vi "RC_Test.vi"() -> ()   [LabVIEW 2013]
uses:
  Data/TypeDefs/DynamixelCycleTracker.ctl
  Data/TypeDefs/Rudder Set Suggestions.ctl
  Data/TypeDefs/HindbrainControlOptions.ctl
  Data/TypeDefs/MotorSetup.ctl
  Data/TypeDefs/DynamixelSetupInfo.ctl
  <vilib>/FPGAPlugInAG/myRIO-1900/niLvFpga_Open_myRIO-1900.vi
  <vilib>/rvi/interface/common/dynamic/niFpgaDynamicAddResources.vi
  <vilib>/rvi/interface/nirviOpenFPGA/nirviOpenFPGA.xnode
  FPGA Bitfiles/AutonomousSailbo_FPGATarget_myRIOPWMDecoder_0snwDOwOU4s.lvbitx
  FPGA_Code/myRIO_PWM_Decoder.vi
  <instrlib>/Dynamixel Motor/Dynamixel Motor.lvlib
panel:
  out "Waveform Chart, Sail 1":dbl(graph)
  out "Waveform Chart, Sail 2":dbl(graph)
  out "error out":errorcluster[](array[cluster])
  in  "Sail 1 Calibration Speed":dbl
  in  "Sail 2 Bound Offset":dbl=800.0
  in  "Sail 1 Bound Offset":dbl=800.0
  in  "Sail 2 Calibration Speed":dbl
  in  "Use Speed\nControl":bool
  out "Position Sail 2":dbl
  out "Position Sail 1":dbl
  out "Calibration loop counter":i32
  in  "Dynamixel Bounds":T1={"Main Dynamixel Set Data"={"Lower Winch Bound (deg)"=0.0, "Upper Winch Bound (deg)"=0.0}, "Rudder Dynamixel Set Data"={"Lower Winch Bound (deg)"=15.0, "Upper Winch Bound (deg)"=60.0}, "Jib Dynamixel Set Data"={"Lower Winch Bound (deg)"=0.0, "Upper Winch Bound (deg)"=0.0}}
  in  "Sail 1 Lower Bound":dbl
  in  "Sail 2 Lower Bound":dbl
  in  "Stop Calibration":bool
  in  "Mode control":T3=enum."RC_control"
  out "Motors IDs Found":u8[](array[numeric])
  out "Commanded rudder value":T4 min=-0.95 max=0.95 scale=1.0..-1.0
  out "Commanded sail value":dbl
  out "Write loop counter":i32
  out "Updated Dynamixel Cycles":T5
  out "Dynamixel Positions (deg)":dbl[](array[numeric])
  out "Read loop counter":i32
  in  "Stop reading":bool
  in  "Stop writing":bool
  in  "VISA resource name":refnum<visa-resource-name>="ASRL3::INSTR"
  # "Read from RC Controller"
  # "Read from Dynamixels"
  # "Check value rudder is being commanded to in position control"
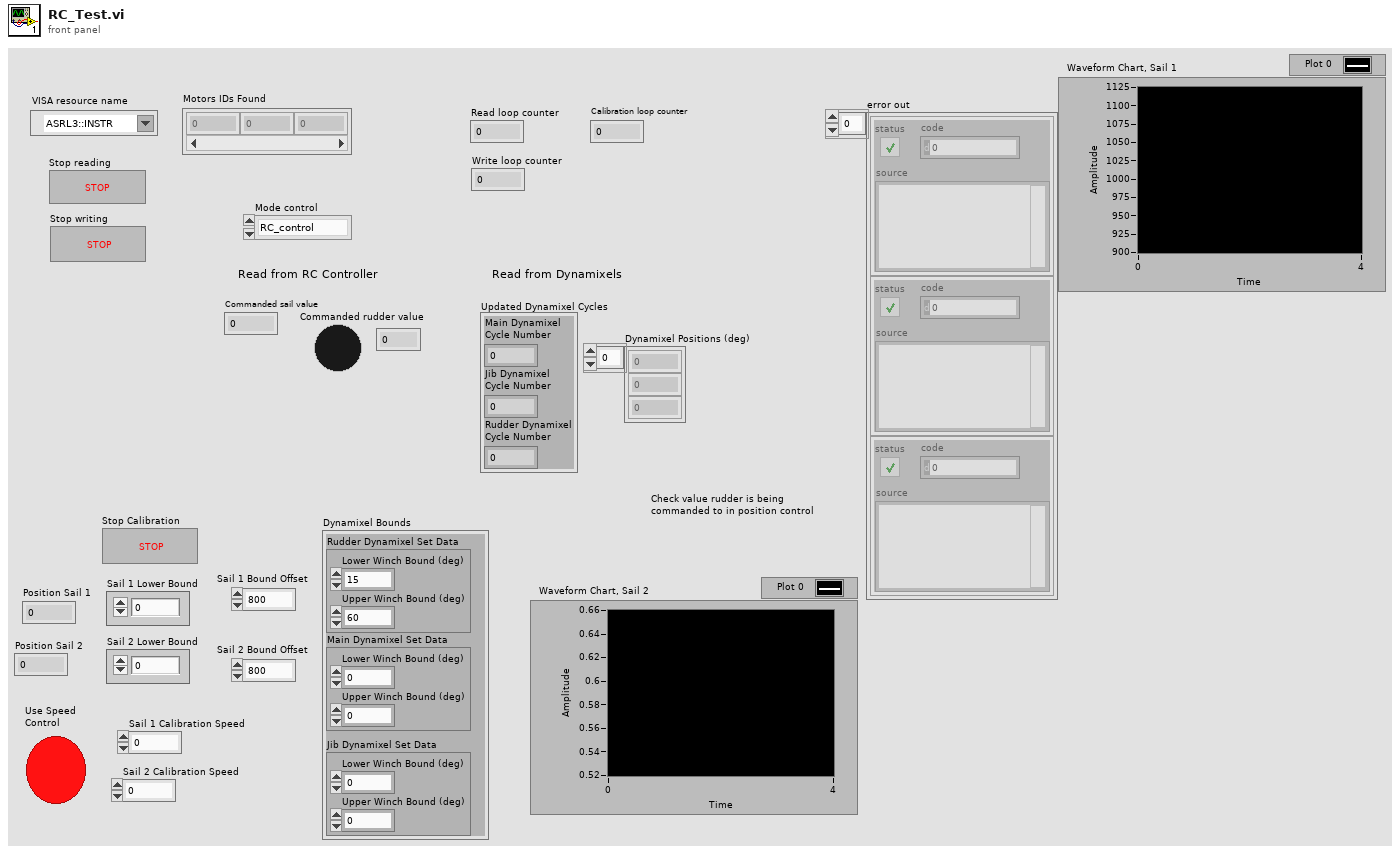
[diagram p1: front panel]
types:
  T1 = typedef "MotorSetup.ctl" = cluster{"Main Dynamixel Set Data":T2, "Rudder Dynamixel Set Data":T2, "Jib Dynamixel Set Data":T2}
  T2 = typedef "DynamixelSetupInfo.ctl" = cluster{"Lower Winch Bound (deg)":dbl, "Upper Winch Bound (deg)":dbl}
  T3 = typedef "HindbrainControlOptions.ctl" = enum16{"code_control", "RC_control", "hand_control"}
  T4 = typedef "Rudder Set Suggestions.ctl" = dbl
  T5 = typedef "DynamixelCycleTracker.ctl" = cluster{"Main Dynamixel\nCycle Number":i32, "Jib Dynamixel\nCycle Number":i32, "Rudder Dynamixel\nCycle Number":i32}
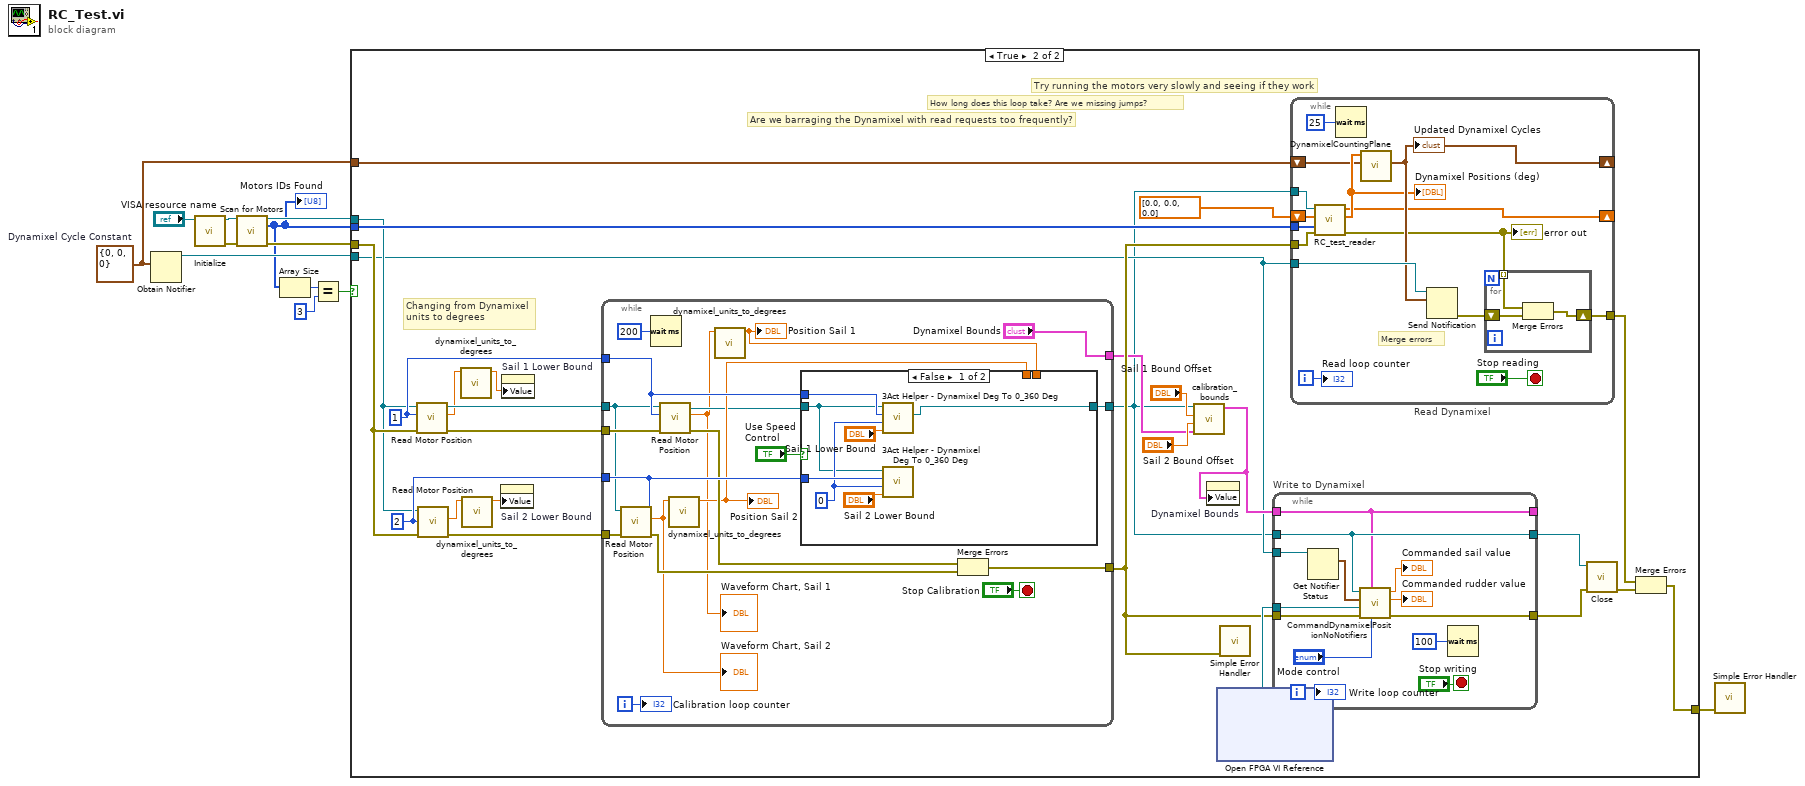
[diagram p0: block diagram]
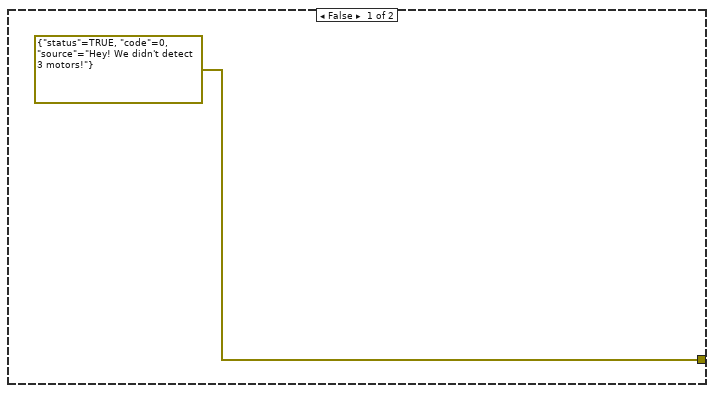
[diagram p2: hidden frame]
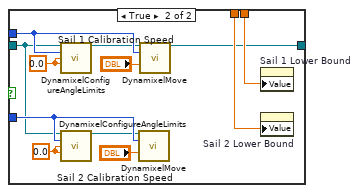
[diagram p3: hidden frame]
diagram:
  w8 = T5 {"Main Dynamixel\nCycle Number"=0, "Jib Dynamixel\nCycle Number"=0, "Rudder Dynamixel\nCycle Number"=0}  # Dynamixel Cycle Constant
  n1 = Obtain Notifier(notification data type=w8) -> (notifier out=w12:refnum<notifier>)  [unwired: 3 in, 2 out]
  n2 = call <instrlib>:"Initialize.vi"("VISA resource name"="VISA resource name") -> ("error out"=w10:errorcluster, "VISA resource name out"=w9:refnum<visa-resource-name>)  [unwired: 9 in]
  n3 = call <instrlib>:"Scan for Motors.vi"("VISA resource name"=w9, "error in (no error)"=w10) -> ("VISA resource name out"=w7:refnum<visa-resource-name>, "Motors IDs Found"=w1:u8[], "error out"=w6:errorcluster)  [unwired: 11 in]
  "Motors IDs Found" <- w1
  n4 = Array Size(array=w1) -> (size(s)=w5:i32)
  n5 = Equal?(x=w5, y=3) -> (x = y?=w4:bool)
  n6 = case shown="True" w4 {
    tunnel: w12 -> [_ w18]
    tunnel: w8 -> [_ w39]
    tunnel: w1 -> [_ w38]
    tunnel: w7 -> [_ w26]
    tunnel: w6 -> [_ w33]
    tunnel: [errorcluster {"status"=TRUE, "code"=0, "source"="Hey! We didn't detect 3 motors!"} ("error IO") w29] -> w2
    frame False {
    }
    frame True {
      w30 = u8 2 ("Motor ID (0)")
      w31 = u8 1 ("Motor ID (0)")
      # "Changing from Dynamixel units to degrees"
      # "Try running the motors very slowly and seeing if they work"
      # "Are we barraging the Dynamixel with read requests too frequently?"
      # "How long does this loop take? Are we missing jumps?"
      n7 = call <instrlib>:"Read Motor Position.vi"("error in (no error)"=w33, "Motor ID (0)"=w31, "VISA resource name"=w26) -> ("error out"=w16:errorcluster, "Position (deg)"=w14:dbl, "VISA resource name out"=w34:refnum<visa-resource-name>)  [unwired: 6 in]
      n8 = call <instrlib>:"Read Motor Position.vi"("error in (no error)"=w33, "Motor ID (0)"=w30, "VISA resource name"=w26) -> ("error out"=w17:errorcluster, "Position (deg)"=w21:dbl)  [unwired: 6 in, 1 out]
      n9 = call "dynamixel_units_to_degrees.vi"("Dynamixel Input"=w14) -> ("Degrees"=w19:dbl)  [unwired: 9 in, 1 out]
      n10 = call "dynamixel_units_to_degrees.vi"("Dynamixel Input"=w21) -> ("Degrees"=w20:dbl)  [unwired: 9 in, 1 out]
      n11 = property on="Sail 2 Lower Bound" class="DigNum (strict)"("Value"=w20) -> ()  [unwired: 2 in, 2 out]
      n12 = property on="Sail 1 Lower Bound" class="DigNum (strict)"("Value"=w19) -> ()  [unwired: 2 in, 2 out]
      n13 = while {
        tunnel: w34 -> [w43]
        tunnel: w31 -> [w55]
        tunnel: w30 -> [w54]
        tunnel: ["Dynamixel Bounds"] -> w22
        tunnel: w17 -> [w53]
        tunnel: [w50] -> w32
        tunnel: w16 -> [w47]
        tunnel: [w45] -> w15
        i -> [w57]
        stop <- "Stop Calibration" stop-if-true
        n14 = call <instrlib>:"Read Motor Position.vi"("error in (no error)"=w53, "Motor ID (0)"=w54, "VISA resource name"=w43) -> ("error out"=w52:errorcluster, "Position (deg)"=w42:dbl)  [unwired: 6 in, 1 out]
        "Waveform Chart, Sail 2" <- w42
        n15 = Wait (ms)(milliseconds to wait=u32 200) -> ()  [unwired: 1 out]
        n16 = call <instrlib>:"Read Motor Position.vi"("error in (no error)"=w47, "Motor ID (0)"=w55, "VISA resource name"=w43) -> ("error out"=w51:errorcluster, "Position (deg)"=w41:dbl, "VISA resource name out"=w46:refnum<visa-resource-name>)  [unwired: 6 in]
        "Waveform Chart, Sail 1" <- w41
        n17 = call "dynamixel_units_to_degrees.vi"("Dynamixel Input"=w42) -> ("Degrees"=w48:dbl)  [unwired: 9 in, 1 out]
        "Position Sail 2" <- w48
        n18 = call "dynamixel_units_to_degrees.vi"("Dynamixel Input"=w41) -> ("Degrees"=w49:dbl)  [unwired: 9 in, 1 out]
        "Position Sail 1" <- w49
        n19 = case shown="False" "Use Speed\nControl" {
          tunnel: w46 -> [w61 w69]
          tunnel: w55 -> [w66 w71]
          tunnel: w54 -> [w65 w77]
          tunnel: w49 -> [_ w75]
          tunnel: w48 -> [_ w73]
          tunnel: [w60 w67] -> w45
          frame False {
            w62 = 0 ("Dynamixel Cycle Number")
            n20 = call "3Act Helper - Dynamixel Deg To 0_360 Deg.vi"("Dynamixel Setpoint In (deg)"="Sail 1 Lower Bound", "Dynamixel Cycle Number"=w62, "Motor ID"=w66, "VISA resource name"=w61) -> ("VISA resource name OUT"=w60:refnum<visa-resource-name>)  [unwired: 5 in, 2 out]
            n21 = call "3Act Helper - Dynamixel Deg To 0_360 Deg.vi"("Dynamixel Setpoint In (deg)"="Sail 2 Lower Bound", "Dynamixel Cycle Number"=w62, "Motor ID"=w65, "VISA resource name"=w61) -> ()  [unwired: 5 in, 3 out]
          }
          frame True {
            w72 = 0.0 ("Clockwise Angle Limit (0 deg)")
            w78 = 0.0 ("Clockwise Angle Limit (0 deg)")
            n22 = call "DynamixelConfigureAngleLimits.vi"("VISA resource name"=w69, "Motor ID (0)"=w71, "Clockwise Angle Limit (0 deg)"=w72, "Counter-Clockwise Angle Limit (300 deg)"=w72) -> ("VISA resource name out"=w68:refnum<visa-resource-name>)  [unwired: 10 in, 1 out]
            n23 = call "DynamixelConfigureAngleLimits.vi"("VISA resource name"=w69, "Motor ID (0)"=w77, "Clockwise Angle Limit (0 deg)"=w78, "Counter-Clockwise Angle Limit (300 deg)"=w78) -> ("VISA resource name out"=w74:refnum<visa-resource-name>)  [unwired: 10 in, 1 out]
            n24 = call "DynamixelMove.vi"("VISA resource name"=w74, "Motor ID (0)"=w77, "Goal Speed (RPM)"="Sail 2 Calibration Speed") -> ()  [unwired: 11 in, 2 out]
            n25 = call "DynamixelMove.vi"("VISA resource name"=w68, "Motor ID (0)"=w71, "Goal Speed (RPM)"="Sail 1 Calibration Speed") -> ("VISA resource name out"=w67:refnum<visa-resource-name>)  [unwired: 11 in, 1 out]
            n26 = property on="Sail 1 Lower Bound" class="DigNum (strict)"("Value"=w75) -> ()  [unwired: 2 in, 2 out]
            n27 = property on="Sail 2 Lower Bound" class="DigNum (strict)"("Value"=w73) -> ()  [unwired: 2 in, 2 out]
          }
        }
        n28 = Merge Errors(w51, w52) -> (w50:errorcluster)
        "Calibration loop counter" <- w57
      }
      n29 = call "calibration_bounds.vi"("Dynamixel Bounds"=w22, "Sail 2 Bound Offset"="Sail 2 Bound Offset", "Sail 1 Bound Offset"="Sail 1 Bound Offset", "VISA resource name in"=w15) -> ("Dynamixel Bounds Out"=w23:T1)  [unwired: 7 in]
      n30 = property on="Dynamixel Bounds" class="Clust (strict)"("Value"=w23) -> ()  [unwired: 2 in, 2 out]
      n31 = xnode "Open FPGA VI Reference"() -> ("FPGA VI Reference Out"=w40:refnum<k20>)  [unwired: 2 in, 1 out]
      n32 = call <vilib>:"Simple Error Handler.vi"("error in (no error)"=w32) -> ()  [unwired: 4 in, 5 out]
      n33 = while "Write to Dynamixel" {
        tunnel: w40 -> [w91]
        tunnel: w15 -> [w84]
        tunnel: w18 -> [w90]
        tunnel: w32 -> [w88]
        tunnel: [w87] -> w27
        tunnel: [w84] -> w28
        tunnel: [w79] -> _
        tunnel: w23 -> [w79]
        i -> [w83]
        stop <- "Stop writing" stop-if-true
        n34 = Get Notifier Status(notifier=w90) -> (current notification=w89:T5)  [unwired: 1 in, 4 out]
        n35 = call "CommandDynamixelPositionNoNotifiers.vi"("Mode control"="Mode control", "Dynamixel Bounds"=w79, "error in"=w88, "FPGA VI Reference In"=w91, "Dynamixel Cycles"=w89, "VISA resource name"=w84) -> ("Error out"=w87:errorcluster, "Commanded rudder value"=→"Commanded rudder value":T4, "Commanded sail value"=→"Commanded sail value":dbl)  [unwired: 3 in]
        n36 = Wait (ms)(milliseconds to wait=u32 100) -> ()  [unwired: 1 out]
        "Write loop counter" <- w83
      }
      n37 = while "Read Dynamixel" {
        tunnel: w15 -> [w105]
        shift-right: [w103] -> _
        shift-left: w39 -> [w95]
        tunnel: w18 -> [w104]
        tunnel: w38 -> [w101]
        tunnel: w32 -> [w106]
        shift-right: [w97] -> _
        shift-left: dbl[] [0.0, 0.0, 0.0] -> [w96]
        tunnel: [w92] -> w35
        i -> [w100]
        stop <- "Stop reading" stop-if-true
        # "Merge errors"
        n38 = call "RC_test_reader.vi"("error in (no error)"=w106, "Motors IDs Found"=w101, "Read positions (dyn)"=w96, "VISA Refnum in"=w105) -> ("error out"=w93:errorcluster[], "Dynamixel Positions (deg)"=w99:dbl[], "Read positions latest (dyn)"=w97:dbl[])  [unwired: 5 in]
        "Dynamixel Positions (deg)" <- w99
        "error out" <- w93
        n39 = Wait (ms)(milliseconds to wait=u32 25) -> ()  [unwired: 1 out]
        n40 = call "DynamixelCountingPlane.vi"("Dynamixel Cycles"=w95, "Dynamixel Read Positions"=w99) -> ("Updated Dynamixle Cycles"=w103:T5)  [unwired: 9 in]
        "Updated Dynamixel Cycles" <- w103
        n41 = Send Notification(notification=w103, notifier=w104) -> (error out=w94:errorcluster)  [unwired: 1 in, 1 out]
        n42 = for {
          shift-right: [w109] -> w92
          shift-left: w94 -> [w108]
          tunnel: w93 -> [w107] mode=indexing
          n43 = Merge Errors(w107, w108) -> (w109:errorcluster)
        }
        "Read loop counter" <- w100
      }
      n44 = call <instrlib>:"Close.vi"("error in (no error)"=w27, "VISA resource name"=w28) -> ("error out"=w37:errorcluster)  [unwired: 9 in]
      n45 = Merge Errors(w35, w37) -> (w29:errorcluster)
    }
  }
  n46 = call <vilib>:"Simple Error Handler.vi"("error in (no error)"=w2) -> ()  [unwired: 4 in, 5 out]
